vi "Set Function a sqrt(dX+c)+b.vi"(0 "VISA resource name":refnum<visa-resource-name>, 1 "Channel unit":string, 5 "Channel":u16(ring) items=["A1"=0, "A2"=1, "A3"=2, "A4"=3, "A5"=4, "A6"=5, "A7"=6, "A8"=7, "A9"=8, "A10"=9, "K1"=200, "K2"=201, "K3"=202, "K4"=203, "FA1"=204, "FA2"=205, "FA3"=206, "FA4"=207], 7 "A coef.":dbl, 9 "B coef.":dbl, 11 "error in (no error)":errorcluster, 12 "C coef.":dbl, 13 "D coef.":dbl) -> (4 "VISA resource name out":refnum<visa-resource-name>, 15 "error out":errorcluster)   [LabVIEW 2017, in "Sefram DAS220.lvlib"]
doc: "Function a*sqrt(dX+c) + b"
uses:
  <instrlib>/Sefram DAS220/Sefram DAS220.lvlib
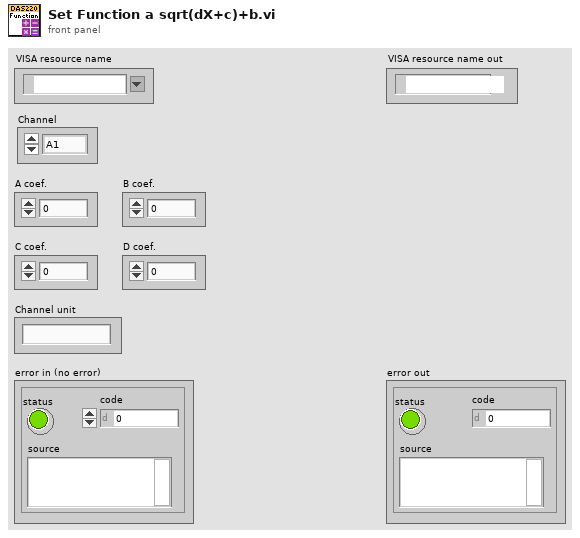
[diagram p1: front panel]
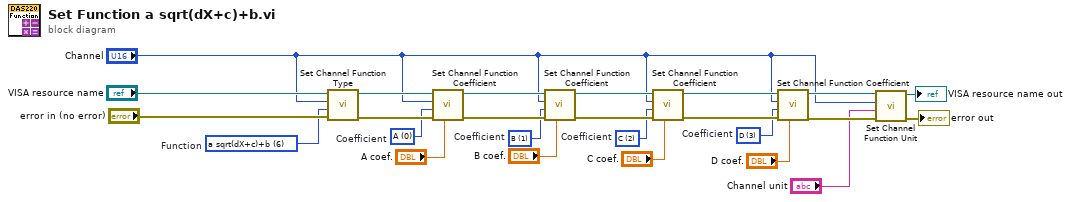
[diagram p0: block diagram]
diagram:
  w2 = u16 6 items=["None", "Change Unit", "aX+b", "a abs(X)+b", "aX2+bX+c", "a ln(X)+b", "a sqrt(dX+c)+b", "a exp(cX)+b", "a(1/X)+b"]  # Function
  w3 = u16 3 items=["A", "B", "C", "D", "X1", "X2", "Y1", "Y2"]  # Coefficient
  w4 = u16 2 items=["A", "B", "C", "D", "X1", "X2", "Y1", "Y2"]  # Coefficient
  w5 = u16 1 items=["A", "B", "C", "D", "X1", "X2", "Y1", "Y2"]  # Coefficient
  w6 = u16 0 items=["A", "B", "C", "D", "X1", "X2", "Y1", "Y2"]  # Coefficient
  n1 = call <instrlib>:"Set Channel Function Type.vi"("error in (no error)"="error in (no error)", "Function"=w2, "Channel"="Channel", "VISA resource name"="VISA resource name") -> ("error out"=w22:errorcluster, "VISA resource name out"=w23:refnum<visa-resource-name>)  [unwired: 6 in]
  n2 = call <instrlib>:"Set Channel Function Coefficient.vi"("Coefficient value"="A coef.", "error in (no error)"=w22, "Coefficient"=w6, "Channel"="Channel", "VISA resource name"=w23) -> ("error out"=w20:errorcluster, "VISA resource name out"=w21:refnum<visa-resource-name>)  [unwired: 5 in]
  n3 = call <instrlib>:"Set Channel Function Coefficient.vi"("Coefficient value"="B coef.", "error in (no error)"=w20, "Coefficient"=w5, "Channel"="Channel", "VISA resource name"=w21) -> ("error out"=w18:errorcluster, "VISA resource name out"=w19:refnum<visa-resource-name>)  [unwired: 5 in]
  n4 = call <instrlib>:"Set Channel Function Coefficient.vi"("Coefficient value"="C coef.", "error in (no error)"=w18, "Coefficient"=w4, "Channel"="Channel", "VISA resource name"=w19) -> ("error out"=w16:errorcluster, "VISA resource name out"=w17:refnum<visa-resource-name>)  [unwired: 5 in]
  n5 = call <instrlib>:"Set Channel Function Coefficient.vi"("Coefficient value"="D coef.", "error in (no error)"=w16, "Coefficient"=w3, "Channel"="Channel", "VISA resource name"=w17) -> ("error out"=w14:errorcluster, "VISA resource name out"=w15:refnum<visa-resource-name>)  [unwired: 5 in]
  n6 = call <instrlib>:"Set Channel Function Unit.vi"("error in (no error)"=w14, "Channel unit"="Channel unit", "Channel"="Channel", "VISA resource name"=w15) -> ("error out"=→"error out":errorcluster, "VISA resource name out"=→"VISA resource name out":refnum<visa-resource-name>)  [unwired: 6 in]
